vi "CC Launch AirMass Calculator.vi"(8 "error in (no error)":errorcluster, 9 "Show Plots?":bool, 10 "Observation List":T1[](array[typedef]), 11 "AirMass program":path) -> (0 "error out":errorcluster, 2 "Air Mass":T7[](array[typedef]), 3 "BlockIDs":string[](array[string]))   [LabVIEW 2024]
uses:
  CC cluster Air Mass Data.ctl
  typedefs/CC cluster Observation.ctl
  CC enum Observation Status.ctl
  Telescope/CC cluster Telescope Offsets.ctl
  typedefs/CC cluster Observation Dither Options.ctl
  typedefs/CC enum Dither Selection.ctl
  typedefs/CC cluster RA and DEC.ctl
panel:
  out "standard error":string
  out "standard output":string
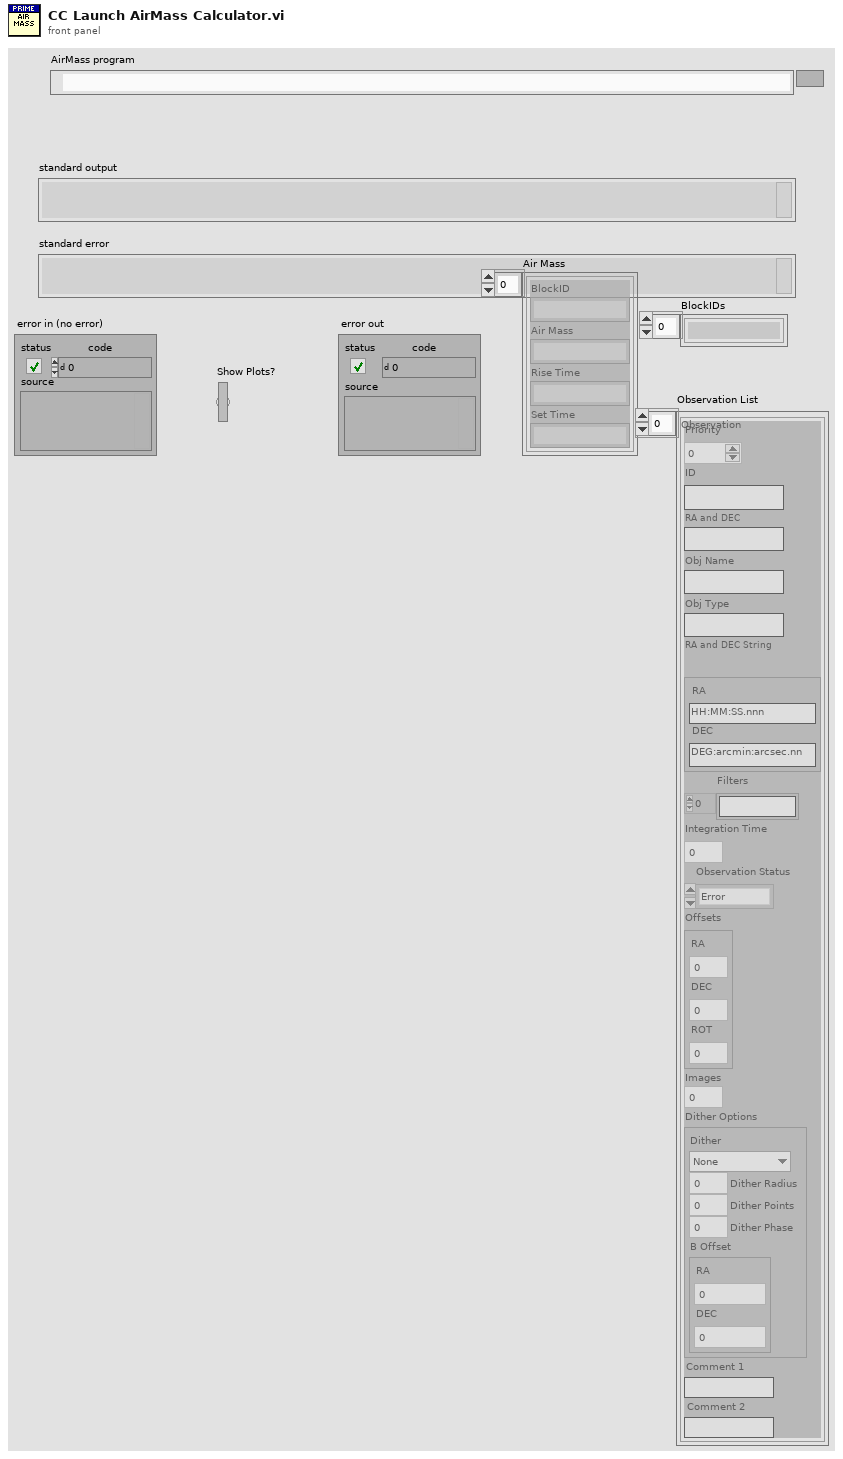
[diagram p1: front panel]
types:
  T1 = typedef "CC cluster Observation.ctl" = cluster{"Priority":i32, "ID":string, "Observer":string, "Obj Name":string, "Obj Type":string, "RA and DEC String":cluster{"RA":string, "DEC":string}, "Filters":string[], "Integration Time":dbl, "Observation Status":T2, "Offsets":T3, "Images":i32, "Dither Options":T4, "Comment 1":string, "Comment 2":string}
  T2 = typedef "CC enum Observation Status.ctl" = enum16{"Ready", "Running", "Done", "Error"}
  T3 = typedef "CC cluster Telescope Offsets.ctl" = cluster{"RA":dbl, "DEC":dbl, "ROT":dbl}
  T4 = typedef "CC cluster Observation Dither Options.ctl" = cluster{"Dither":T5, "Dither Radius":dbl, "Dither Points":i32, "Dither Phase":dbl, "B Offset":T6}
  T5 = typedef "CC enum Dither Selection.ctl" = enum16{"None", "Circle", "Random", "ABBA"}
  T6 = typedef "CC cluster RA and DEC.ctl" = cluster{"RA":dbl, "DEC":dbl}
  T7 = typedef "CC cluster Air Mass Data.ctl" = cluster{"BlockID":string, "Air Mass":string, "Rise Time":string, "Set Time":string}
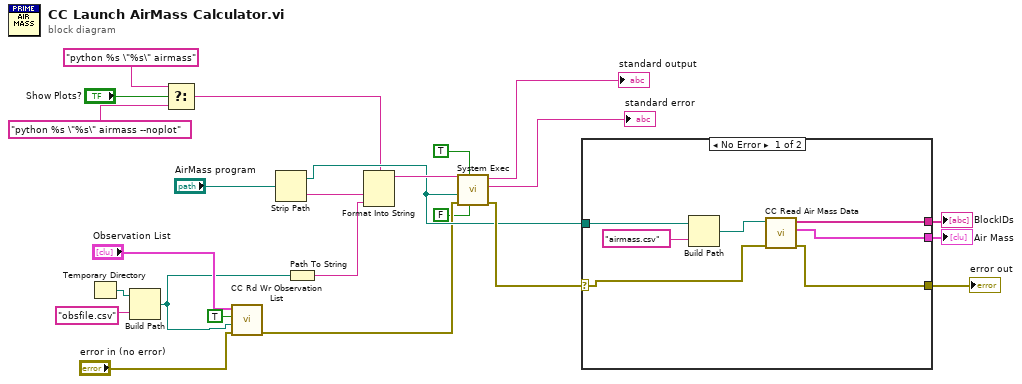
[diagram p0: block diagram]
diagram:
  n1 = Temporary Directory() -> (w12:path)
  n2 = Build Path(base path=w12, name or relative path="obsfile.csv") -> (appended path=w6:path)
  n3 = Select(t="python %s \"%s\" airmass" ("format string"), s="Show Plots?", f="python %s \"%s\" airmass --noplot" ("format string")) -> (s? t:f=w2:string)
  n4 = call "CC Rd Wr Observation List.vi"("error in (no error)"="error in (no error)", "filepath"=w6, "Write? (F:Read)"=TRUE, "Observation List"="Observation List") -> ("error out"=w7:errorcluster)  [unwired: 4 in, 3 out]
  n5 = Strip Path(path="AirMass program") -> (stripped path=w16:path, name=w23:string)
  n6 = Path To String(path=w6) -> (string=w22:string)
  n7 = Format Into String(format string=w2, w23, w22) -> (resulting string=w21:string)  [unwired: 2 in, 1 out]
  n8 = call <vilib>:"System Exec.vi"("run minimized? (F)"=FALSE, "wait until completion? (T)"=TRUE, "error in (no error)"=w7, "working directory"=w16, "command line"=w21) -> ("error out"=w17:errorcluster, "standard error"=→"standard error":string, "standard output"=→"standard output":string)  [unwired: 3 in, 1 out]
  n9 = case shown="No Error" w17 {
    selector: w17 -> [w28 w32]
    tunnel: w16 -> [w31 _]
    tunnel: [w27 w32] -> w15
    tunnel: [w26 _] -> w13
    tunnel: [w25 _] -> w14
    frame No Error {
      n10 = Build Path(base path=w31, name or relative path="airmass.csv") -> (appended path=w29:path)
      n11 = call "CC Read Air Mass Data.vi"("error in (no error)"=w28, "file path (dialog if empty)"=w29) -> ("error out"=w27:errorcluster, "Air Mass"=w25:T7[], "BlockIDs"=w26:string[])  [unwired: 7 in]
    }
    frame Error {
    }
  }
  "error out" <- w15
  "Air Mass" <- w14
  "BlockIDs" <- w13
